vi "Simple Tester.vi"() -> ()   [LabVIEW 2016, in "Simple Tester.lvclass"]
doc: "This is the Simple Tester VI. It:\n - Tests the functionality of the Error Manager module\n - Serves as an environment in which new features or bug fixes can be tested\n - Serves as an introduction and demonstration of how to use the Error Manager"
uses:
  Simple Tester.lvclass
  Error Manager/Error Manager.lvlib
  Dummy Error Message Length (enum).ctl
panel:
  out "Simple Tester Settings Filepath":path
  in  "Random Error Message Length":T1=enum."Medium (Up to 1,000 characters)"
  in  "Use random error codes and messages?":bool=TRUE
  out "Error Out":errorcluster
  in  "Error Code":i32=-1
  in  "Show Call Chain?":bool=TRUE
  in  "Error Message":string="Dummy error (testing)"
  in  "Error?":bool
  in  "Stop Tester":bool
  out "Loop Iteration":i32
  in  "Generate Error":bool
  # "Simple Tester\n\nInstructions\n1. Run the VI\n2. Press 'Generate Error' to generate an error.\n    - If you wish, you can change the Error code, the Error Message, and whether the call chain is to be contained in the error message or not.\n3. Press the 'No error/Error' button to bring up the Error Manager GUI (in other words, to show the Front Panel of the Error Handler asynchronous module). This is analogous to how a user would press bring up the Error Manager GUI in a real application that uses the Error Handler.\n4. Inspect the Error Manager GUI. Use the buttons/controls/indicators available in the Error Manager GUI.\n    - Navigate to or open the Error Log text file"
  # "Press this button to view the Error Manager main window"
  # "This button simulates an \"Error/No error\" button on the Main GUI VI of the host application. Such a button is typically part on the application's status bar (top or bottom bar). You can copy this button into the GUI of the host app if you wish."
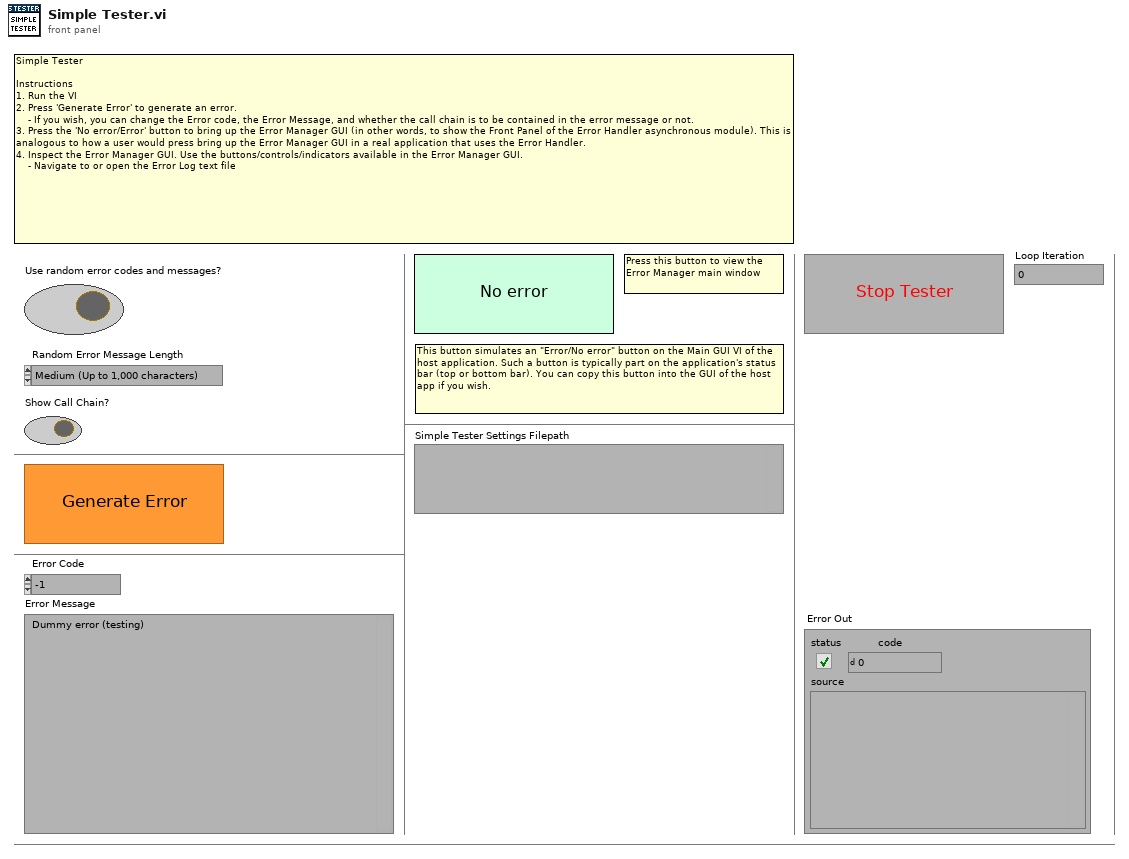
[diagram p1: front panel]
types:
  T1 = typedef "Simple Tester.lvclass/Dummy Error Message Length (enum).ctl" = enum16{"Short (Up to 100 characters)", "Medium (Up to 1,000 characters)", "Long (Up to 10,000 characters)"}
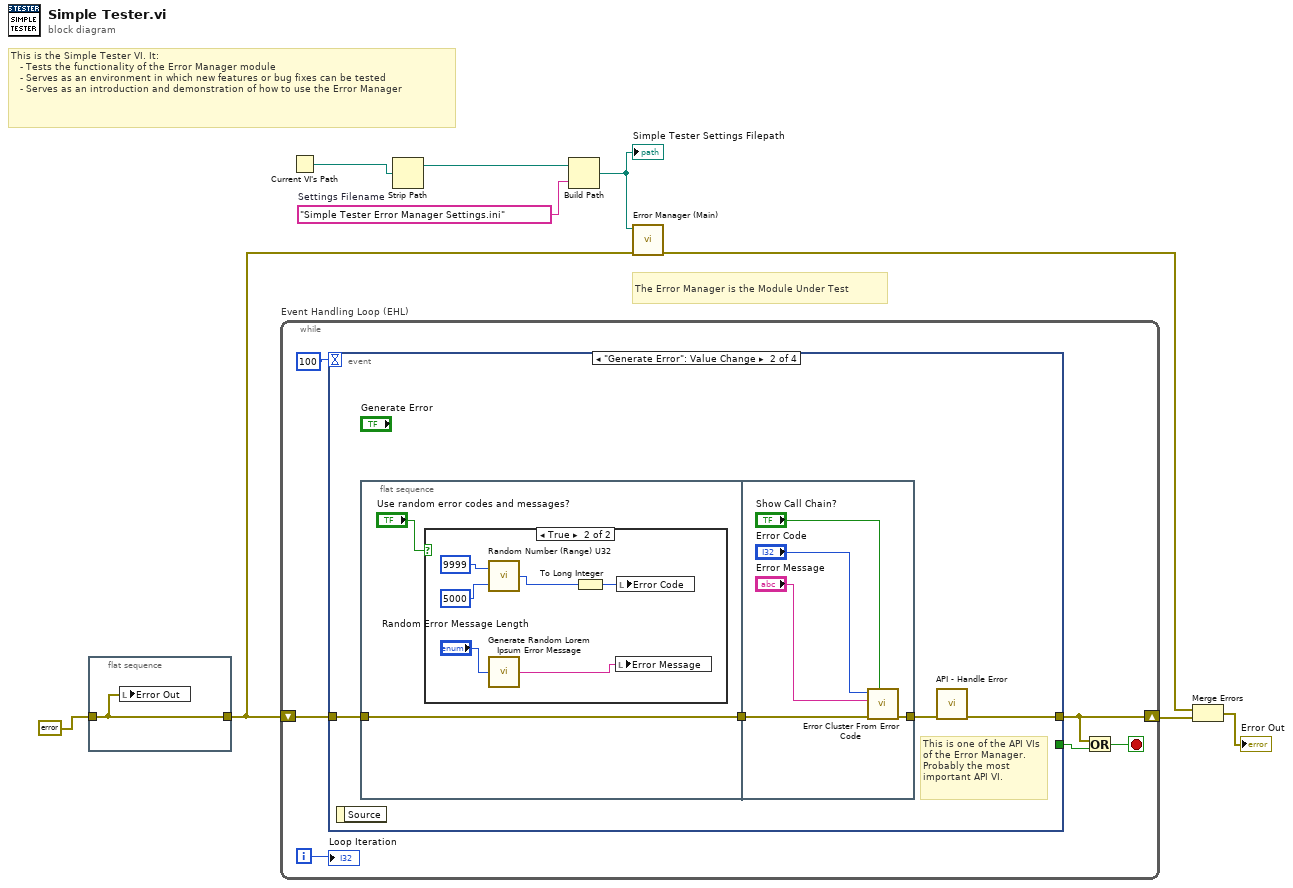
[diagram p0: block diagram]
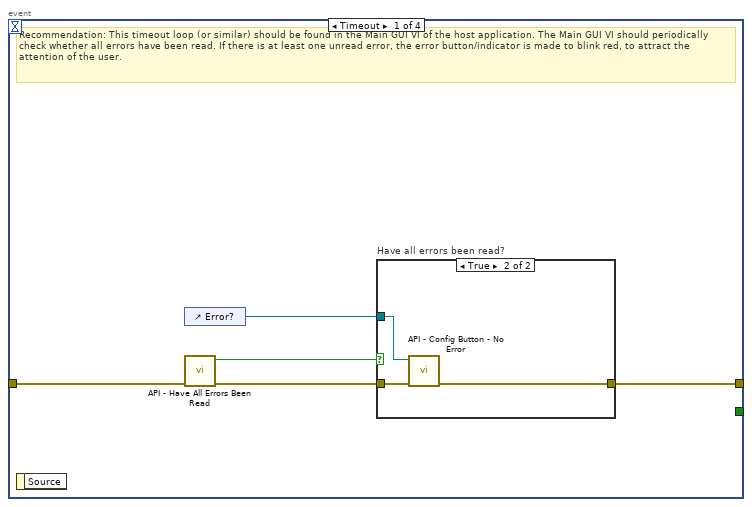
[diagram p2: hidden frame]
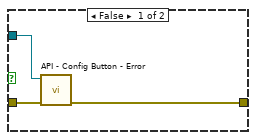
[diagram p3: hidden frame]
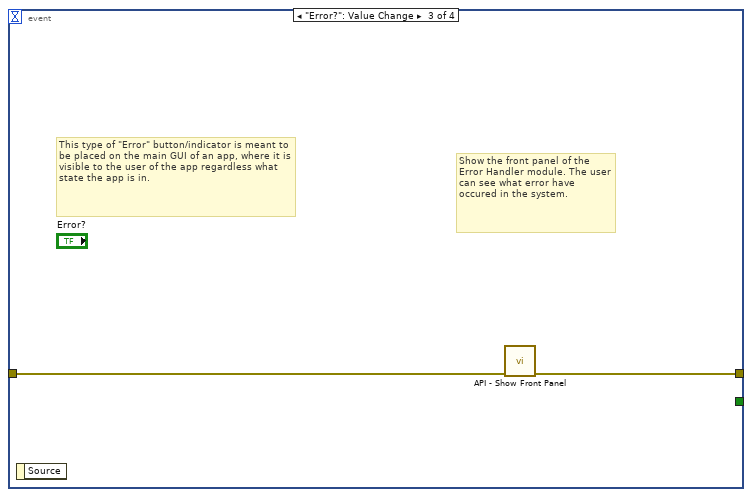
[diagram p5: hidden frame]
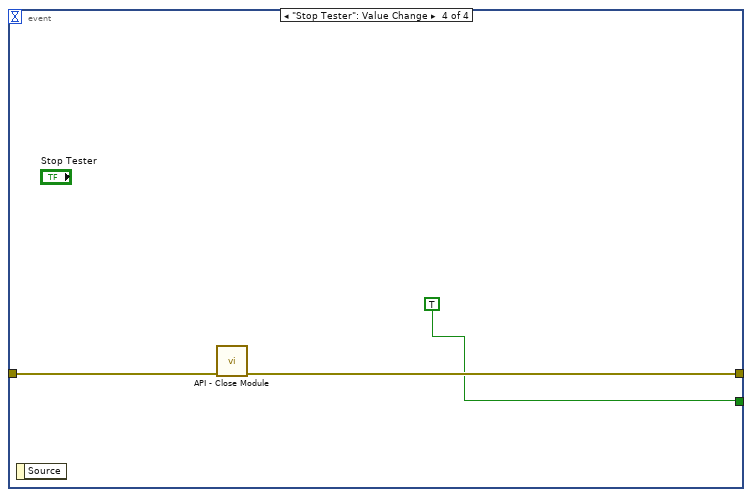
[diagram p6: hidden frame]
diagram:
  w2 = "Simple Tester Error Manager Settings.ini"  # Settings Filename
  # "The Error Manager is the Module Under Test"
  # "This is the Simple Tester VI. It:\n   - Tests the functionality of the Error Manager module\n   - Serves as an environment in which new features or bug fixes can be tested\n   - Serves as an introduction and demonstration of how to use the Error Manager"
  n1 = flat-sequence {
    tunnel: [w10] -> w6
    tunnel: errorcluster {"status"=FALSE, "code"=0, "source"=""} ("error constant") -> [w10]
    frame #0 {
      n2 = local write "Error Out"(w10) -> ()
    }
  }
  n3 = while "Event Handling Loop (EHL)" {
    shift-right: [w13] -> w8
    shift-left: w6 -> [w14]
    i -> [w16]
    stop <- w11 stop-if-true
    n4 = event shown="[1] \"Generate Error\": Value Change" {
      selector: _ -> [_ _ _ _]
      dyn-events: _ -> [_ _ _ _]
      timeout: 100 -> [_ _ _ _]
      tunnel: w14 -> [w21 w29 w46 w48]
      tunnel: [w19 w31 w45 w49] -> w13
      tunnel: [_ _ _ TRUE] -> w12
      event Timeout {
        # "Recommendation: This timeout loop (or similar) should be found in the Main GUI VI of the host application. The Main GUI VI should periodically check whether all errors have been read. If there is at least one unread error, the error button/indicator is made to blink red, to attract the attention of the user."
        n5 = event-data() -> ()  [unwired: 1 in, 1 out]
        n6 = control-ref of="Error?"() -> (w17:refnum<vi>)
        n7 = call "API - Have All Errors Been Read.vi"("error in"=w21) -> ("error out"=w20:errorcluster, "Have All Errors Been Read?"=w18:bool)  [unwired: 9 in]
        n8 = case "Have all errors been read?" shown="True" w18 {
          tunnel: [w22 w26] -> w19
          tunnel: w20 -> [w23 w27]
          tunnel: w17 -> [w24 w25]
          frame False {
            n9 = call "API - Config Button - Error.vi"("error in"=w23, "Error Button"=w24) -> ("error out"=w22:errorcluster)  [unwired: 9 in]
          }
          frame True {
            n10 = call "API - Config Button - No Error.vi"("error in"=w27, "Error Button"=w25) -> ("error out"=w26:errorcluster)  [unwired: 9 in]
          }
        }
      }
      event "Generate Error": Value Change {
        # "This is one of the API VIs of the Error Manager. Probably the most important API VI."
        n11 = event-data() -> ()  [unwired: 1 in, 1 out]
        n12 = flat-sequence {
          tunnel: w29 -> [w33]
          tunnel: [w33] -> w28
          tunnel: [w44] -> w30
          tunnel: w28 -> [w43]
          frame #0 {
            n13 = case shown="True" "Use random error codes and messages?" {
              frame False {
              }
              frame True {
                n14 = call "Random Number (Range) U32.vi"("lower bound"=u32 5000 ("lower bound (0)"), "upper bound"=u32 9999 ("upper bound (100)")) -> ("number"=w35:u32)
                n15 = call "Generate Random Lorem Ipsum Error Message.vi"("Dummy Error Message Length"="Random Error Message Length") -> ("Random Lorem Ipsum Error Message (dummy error message)"=w38:string)
                n16 = To Long Integer(number=w35) -> (32bit integer=w34:i32)
                n17 = local write "Error Message"(w38) -> ()
                n18 = local write "Error Code"(w34) -> ()
              }
            }
          }
          frame #1 {
            n19 = call <vilib>:"Error Cluster From Error Code.vi"("show call chain? (False)"="Show Call Chain?", "error in (no error)"=w43, "error message (\"\")"="Error Message", "error code (0)"="Error Code") -> ("error out"=w44:errorcluster)  [unwired: 5 in]
          }
        }
        n20 = call "API - Handle Error.vi"("error in"=w30) -> ("error out"=w31:errorcluster)  [unwired: 10 in]
      }
      event "Error?": Value Change {
        # "This type of \"Error\" button/indicator is meant to be placed on the main GUI of an app, where it is visible to the user of the app regardless what state the app is in."
        # "Show the front panel of the Error Handler module. The user can see what error have occured in the system."
        n21 = event-data() -> ()  [unwired: 1 in, 1 out]
        n22 = call "API - Show Front Panel.vi"("error in"=w46) -> ("error out"=w45:errorcluster)  [unwired: 10 in]
      }
      event "Stop Tester": Value Change {
        n23 = event-data() -> ()  [unwired: 1 in, 1 out]
        n24 = call "API - Close Module.vi"("error in"=w48) -> ("error out"=w49:errorcluster)  [unwired: 10 in]
      }
    }
    n25 = Or(x=w13, y=w12) -> (x .or. y?=w11:bool)
    "Loop Iteration" <- w16
  }
  n26 = Current VI's Path() -> (path=w4:path)
  n27 = Strip Path(path=w4) -> (stripped path=w3:path)  [unwired: 1 out]
  n28 = Build Path(base path=w3, name or relative path=w2) -> (appended path=w1:path)
  "Simple Tester Settings Filepath" <- w1
  n29 = call "Error Manager (Main).vi"("Error In"=w6, "Settings Filepath"=w1) -> ("Error Out"=w9:errorcluster)  [unwired: 9 in]
  n30 = Merge Errors(w9, w8) -> (→"Error Out":errorcluster)
